vi "lab1.vi"() -> ()   [LabVIEW 2026]
panel:
  out "Waveform Chart":dbl(graph)
  out "Thermometer":dbl(slide) scale=0.0..100.0
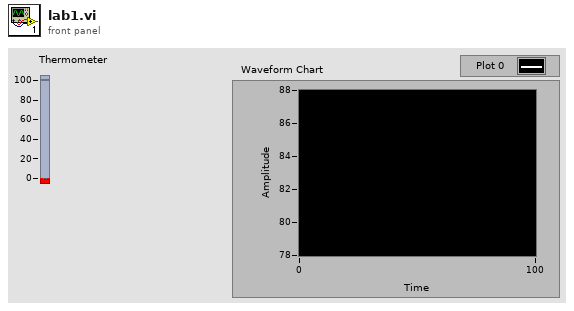
[diagram p1: front panel]
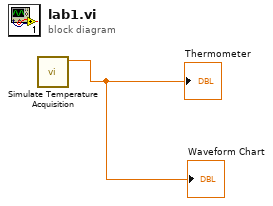
[diagram p0: block diagram]
diagram:
  n1 = call "Simulate Temperature Acquisition.vi"() -> ("temperature"=→"Thermometer" →"Waveform Chart":dbl)  [unwired: 11 in]
